vi "SigArrayTweak.vi"(0 "Signal IN":refnum<k7>, 2 "Style":i32(ring) items=["SigTweakStyleReset", "SigTweakStyleContinue", "SigTweakStyleScale"], 5 "Cycles":i32, 7 "Sample Rate":dbl, 9 "Signal Array":dbl[](array[numeric]), 11 "error in":errorcluster) -> (4 "Signal OUT":refnum<k7>, 15 "error out":errorcluster)   [LabVIEW 2016]
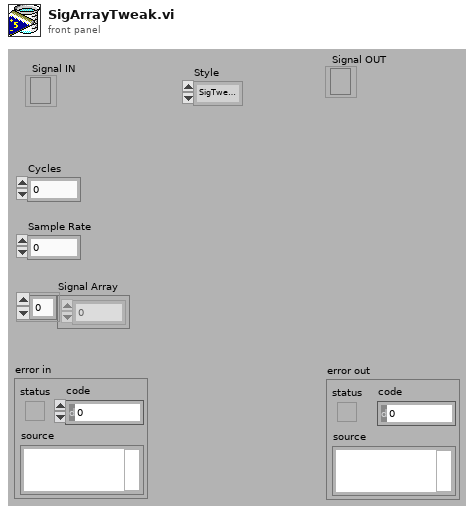
[diagram p1: front panel]
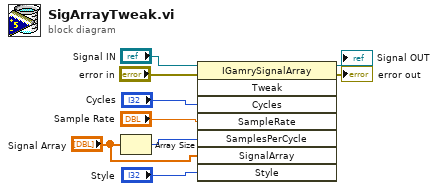
[diagram p0: block diagram]
diagram:
  n1 = Array Size(array="Signal Array") -> (size(s)=w3:i32)
  n2 = invoke class="IGamrySignalArray" method="Tweak"(reference="Signal IN", error in="error in", "Cycles"="Cycles", "SampleRate"="Sample Rate", "SamplesPerCycle"=w3, "SignalArray"="Signal Array", "Style"="Style") -> (reference out=→"Signal OUT":refnum<k7>, error out=→"error out":errorcluster)  [unwired: 1 in, 6 out]
